vi "Sampling Rate Example.vi"() -> ()   [LabVIEW 2009]
uses:
  <vilib>/DAQmx/configure/timing.llb/DAQmx Timing (Sample Clock).vi
  <vilib>/DAQmx/create/channels.llb/DAQmx Create Channel (AI-Voltage-Basic).vi
  <vilib>/DAQmx/write.llb/DAQmx Write (Analog 1D DBL 1Chan NSamp).vi
  <vilib>/DAQmx/create/channels.llb/DAQmx Create Channel (AO-Voltage-Basic).vi
  <vilib>/measure/maspectr.llb/FFT Power Spectrum for 1 Chan.vi
  <vilib>/DAQmx/read.llb/DAQmx Read (Analog Wfm 1Chan NSamp).vi
  <vilib>/measure/NI_MAPro.lvlib
  <vilib>/Analysis/NI_AALBase.lvlib
  Program Files/National Instruments/LabVIEW 2009/resource/objmgr/daqmx.rc
panel:
  in  "DAQmx Device Name":tag="Dev1"
  in  "Analog Output Frequency (Hz)":dbl(knob)=500.0 min=100.0 max=10000.0 scale=100.0..5000.0
  in  "Analog Input Frequency (Hz)":dbl(knob)=1500.0 min=100.0 max=10000.0 scale=100.0..5000.0
  in  "stop":bool
  out "Frequency Domain Data":cluster{"f0":dbl, "df":dbl, "magnitude":dbl[]}(graph)={"f0"=0.0, "df"=50.0, "magnitude"=[]}
  out "Time Domain Data":waveform(dbl)(graph)={"t0"=timestamp(3288286244.6907215 s since 1904-01-01), "dt"=0.00019999999999999998, "Y"=[], "attributes"=variant("NI_ChannelName"=variant(string "cDAQ1Mod2/ai3"), "NI_UnitDescription"=variant(string "Volts"))}
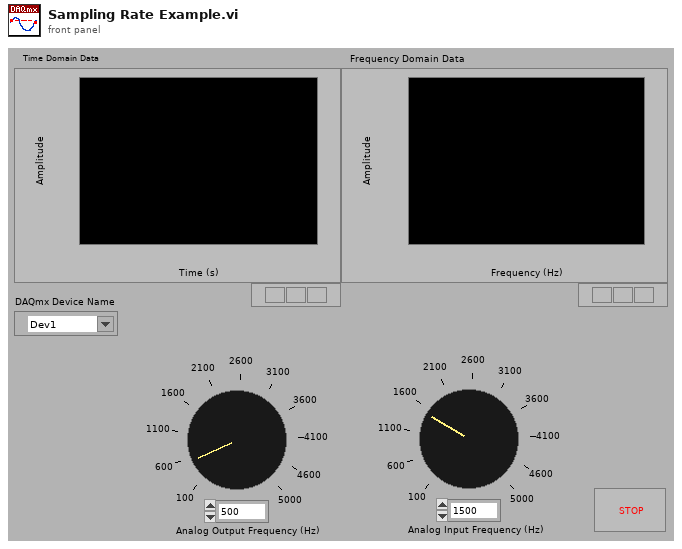
[diagram p1: front panel]
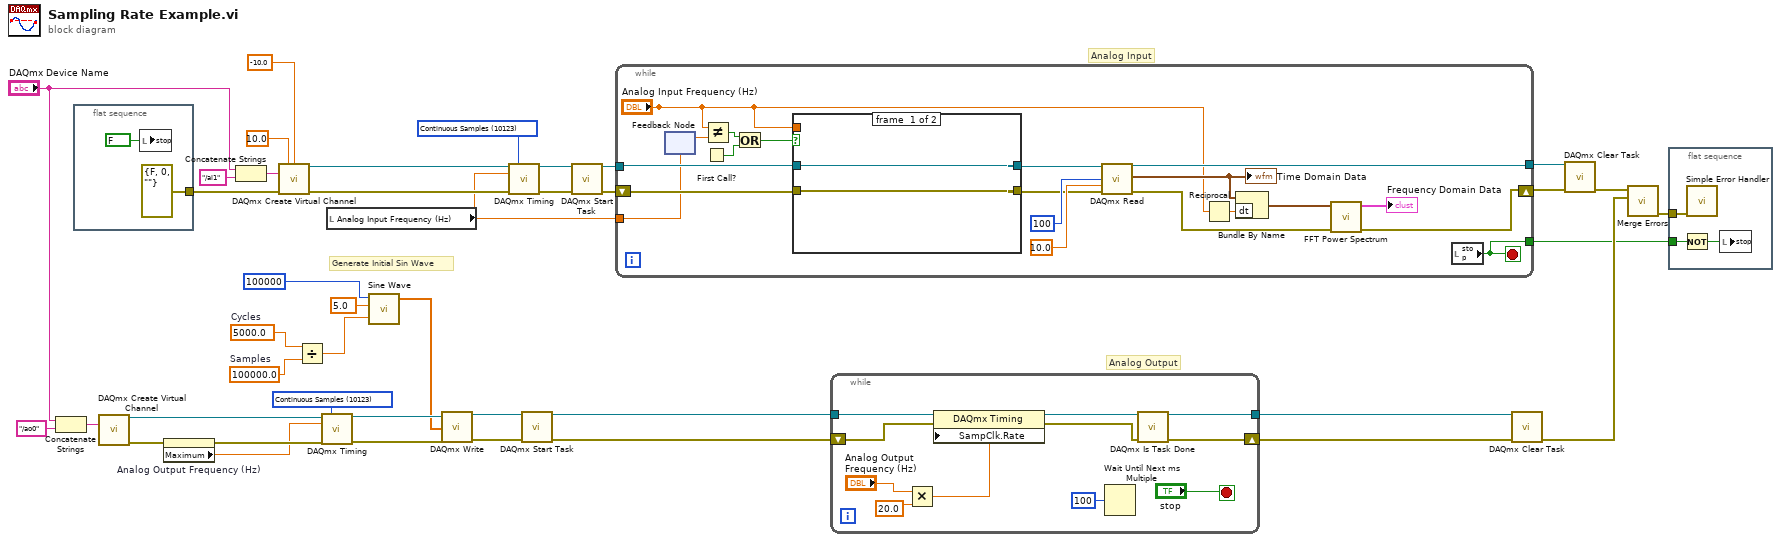
[diagram p0: block diagram]
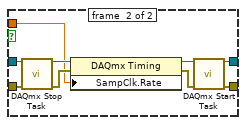
[diagram p2: hidden frame]
diagram:
  w28 = 5000.0  # Cycles
  w30 = 100000.0  # Samples
  w33 = 10123 items=["Finite Samples"=10178, "Continuous Samples"=10123] ("sample mode")
  w35 = 10123 items=["Finite Samples"=10178, "Continuous Samples"=10123] ("sample mode")
  # "Analog Output"
  # "Analog Input"
  # "Generate Initial Sin Wave"
  n1 = Concatenate Strings("DAQmx Device Name", "/ao0" ("string")) -> (w4:string)
  n2 = flat-sequence {
    tunnel: [errorcluster {"status"=FALSE, "code"=0, "source"=""} ("error in")] -> w9
    frame #0 {
      n3 = local write "stop"(FALSE ("stop")) -> ()
    }
  }
  n4 = call-poly <vilib>:"DAQmx Create Virtual Channel.vi"("physical channels"=w4) -> ("task out"=w21:refnum<k21>, "error out"=w19:errorcluster)  [unwired: 13 in]
  n5 = property on="Analog Output Frequency (Hz)" class="Knob (strict)"(error in=w19) -> (error out=w20:errorcluster, "Maximum"=w18:dbl)  [unwired: 1 in, 1 out]
  n6 = Concatenate Strings("DAQmx Device Name", "/ai1" ("string")) -> (w6:string)
  n7 = call-poly <vilib>:"DAQmx Create Virtual Channel.vi"("maximum value"=10.0, "minimum value"=-10.0, "physical channels"=w6, "error in"=w9) -> ("task out"=w39:refnum<k21>, "error out"=w3:errorcluster)  [unwired: 10 in]
  n8 = Divide(x=w28, y=w30) -> (x/y=w29:dbl)
  n9 = call-poly <vilib>:"DAQmx Timing.vi"("task/channels in"=w21, "sample mode"=w33, "rate"=w18, "error in"=w20) -> ("task out"=w32:refnum<k21>, "error out"=w31:errorcluster)  [unwired: 10 in]
  n10 = local read "Analog Input Frequency (Hz)"() -> (w2:dbl)
  n11 = call <vilib>:"Sine Wave.vi"("samples"=100000, "amplitude"=5.0, "frequency"=w29) -> ("sine wave"=w25:dbl[])  [unwired: 2 in, 2 out]
  n12 = call-poly <vilib>:"DAQmx Write.vi"("task/channels in"=w32, "data"=w25, "error in"=w31) -> ("task out"=w17:refnum<k21>, "error out"=w16:errorcluster)  [unwired: 10 in, 1 out]
  n13 = call-poly <vilib>:"DAQmx Timing.vi"("task/channels in"=w39, "sample mode"=w35, "rate"=w2, "error in"=w3) -> ("task out"=w22:refnum<k21>, "error out"=w38:errorcluster)  [unwired: 10 in]
  n14 = call <vilib>:"DAQmx Start Task.vi"("task/channels in"=w17, "error in"=w16) -> ("task out"=w24:refnum<k21>, "error out"=w23:errorcluster)  [unwired: 12 in]
  n15 = call <vilib>:"DAQmx Start Task.vi"("task/channels in"=w22, "error in"=w38) -> ("task out"=w37:refnum<k21>, "error out"=w36:errorcluster)  [unwired: 12 in]
  n16 = while {
    tunnel: w37 -> [w54]
    tunnel: [w61] -> w13
    tunnel: w2 -> [w45]
    tunnel: [w44] -> w1
    shift-right: [w60] -> w14
    shift-left: w36 -> [w51]
    stop <- w44 stop-if-true
    n17 = feedback #1(w45) -> (w50:dbl)
    n18 = First Call?() -> (First Call?: T/F=w46:bool)
    n19 = Not Equal?(x="Analog Input Frequency (Hz)", y=w50) -> (x != y?=w49:bool)
    n20 = Or(x=w49, y=w46) -> (x .or. y?=w47:bool)
    n21 = case shown="True" w47 {
      tunnel: w54 -> [w65 w70]
      tunnel: w51 -> [w64 w69]
      tunnel: [w65 w68] -> w53
      tunnel: [w64 w67] -> w52
      tunnel: "Analog Input Frequency (Hz)" -> [_ w66]
      frame #0 {
      }
      frame #1 {
        n22 = call <vilib>:"DAQmx Stop Task.vi"("task/channels in"=w70, "error in"=w69) -> ("task out"=w72:refnum<k21>, "error out"=w71:errorcluster)  [unwired: 12 in]
        n23 = property class="DAQmx Timing"(reference=w72, error in=w71, "SampClk.Rate"=w66) -> (reference out=w74:refnum<k21>, error out=w73:errorcluster)
        n24 = call <vilib>:"DAQmx Start Task.vi"("task/channels in"=w74, "error in"=w73) -> ("task out"=w68:refnum<k21>, "error out"=w67:errorcluster)  [unwired: 12 in]
      }
    }
    n25 = call-poly <vilib>:"DAQmx Read.vi"("task/channels in"=w53, "number of samples per channel"=100, "timeout"=10.0, "error in"=w52) -> ("task out"=w61:refnum<k21>, "data"=w58:waveform(dbl), "error out"=w55:errorcluster)  [unwired: 9 in]
    "Time Domain Data" <- w58
    n26 = Reciprocal(x="Analog Input Frequency (Hz)") -> (1/x=w57:dbl)
    n27 = Bundle By Name(cluster=w58, "dt"=w57) -> (w56:waveform(dbl))
    n28 = call-poly <vilib>:"FFT Power Spectrum.vi"("error in (no error)"=w55, "time signal"=w56) -> ("error out"=w60:errorcluster, "power spectrum"=→"Frequency Domain Data":cluster{"f0":dbl, "df":dbl, "magnitude":dbl[]})  [unwired: 6 in, 2 out]
    n29 = local read "stop"() -> (w44:bool)
  }
  n30 = while {
    tunnel: w24 -> [w84]
    shift-right: [w78] -> w34
    shift-left: w23 -> [w83]
    tunnel: [w79] -> w15
    stop <- "stop" stop-if-true
    n31 = Multiply(x="Analog Output Frequency (Hz)", y=20.0) -> (x*y=w81:dbl)
    n32 = property class="DAQmx Timing"(reference=w84, error in=w83, "SampClk.Rate"=w81) -> (reference out=w80:refnum<k21>, error out=w77:errorcluster)
    n33 = Wait Until Next ms Multiple(millisecond multiple=u32 100) -> ()  [unwired: 1 out]
    n34 = call <vilib>:"DAQmx Is Task Done.vi"("task/channels in"=w80, "error in"=w77) -> ("task out"=w79:refnum<k21>, "error out"=w78:errorcluster)  [unwired: 11 in, 1 out]
  }
  n35 = call <vilib>:"DAQmx Clear Task.vi"("task in"=w15, "error in"=w34) -> ("error out"=w11:errorcluster)  [unwired: 13 in]
  n36 = call <vilib>:"DAQmx Clear Task.vi"("task in"=w13, "error in"=w14) -> ("error out"=w12:errorcluster)  [unwired: 13 in]
  n37 = call <vilib>:"Merge Errors.vi"("error in 2 (no error)"=w11, "error in 1 (no error)"=w12) -> ("error out"=w10:errorcluster)  [unwired: 5 in]
  n38 = flat-sequence {
    tunnel: w10 -> [w88]
    tunnel: w1 -> [w86]
    frame #0 {
      n39 = Not(x=w86) -> (.not. x?=w87:bool)
      n40 = call <vilib>:"Simple Error Handler.vi"("error in (no error)"=w88) -> ()  [unwired: 4 in, 5 out]
      n41 = local write "stop"(w87) -> ()
    }
  }
